vi "MeasureSinglePointAndStep.vi"(7 "SMU":T2, 8 "Error In":errorcluster, 9 "Source Value":dbl, 10 "Measure Function":T1, 11 "Keithley 2602 In":refnum<visa-resource-name>) -> (0 "Error Out":errorcluster, 2 "Reading":dbl, 3 "Keithley 2602 Out":refnum<visa-resource-name>)   [LabVIEW 2012, in "Keithley-2602.lvlib"]
uses:
  Keithley-2602.lvlib
  Controls/SMU.ctl
  Controls/MeasureFunction.ctl
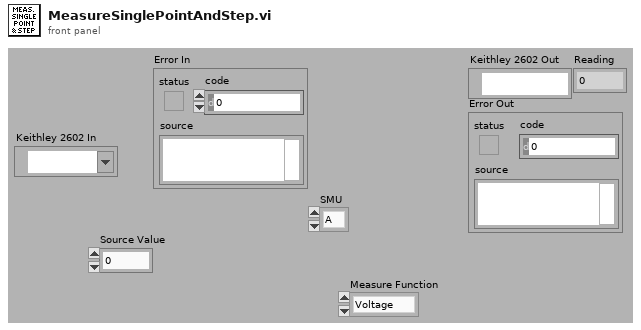
[diagram p1: front panel]
types:
  T1 = typedef "Keithley-2602.lvlib/MeasureFunction.ctl" = enum16{"Voltage", "Current", "Resistance", "Power"}
  T2 = typedef "Keithley-2602.lvlib/SMU.ctl" = enum16{"A", "B"}
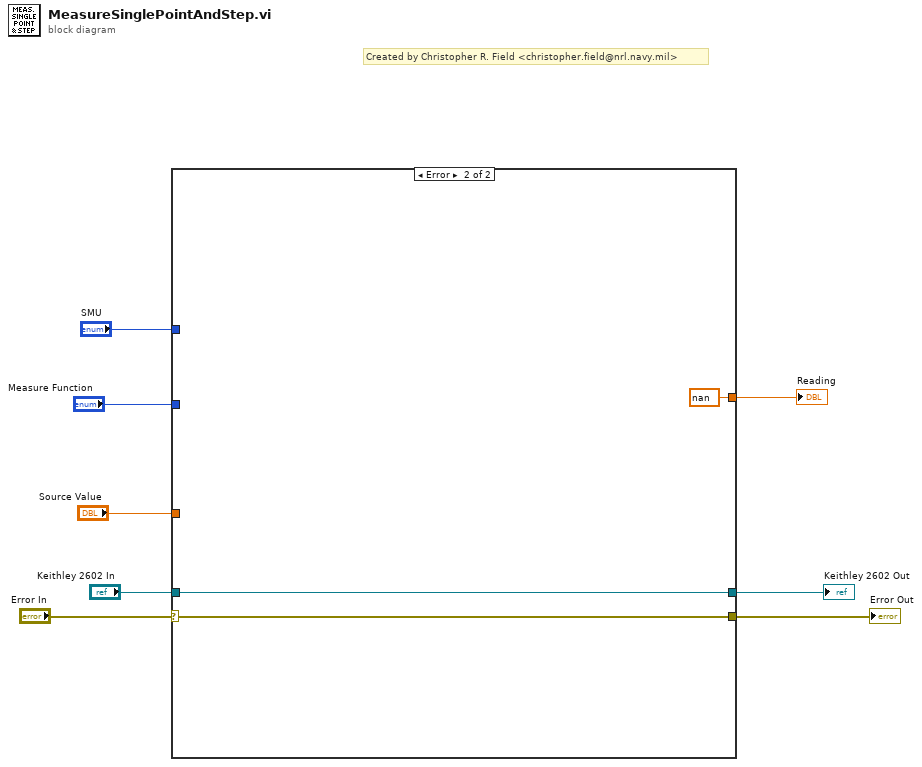
[diagram p0: block diagram]
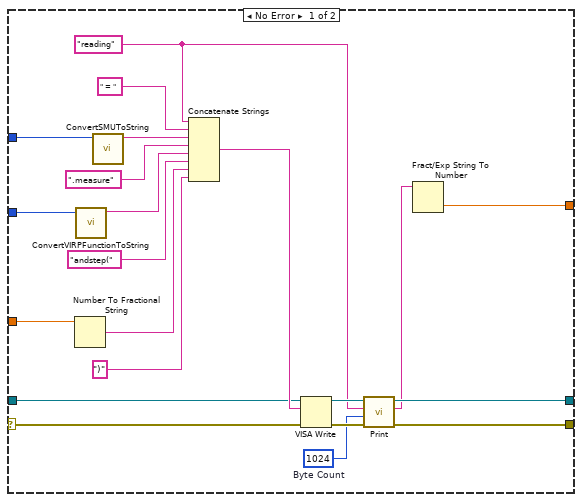
[diagram p2: hidden frame]
diagram:
  # "Created by Christopher R. Field <christopher.field@nrl.navy.mil>"
  n1 = case shown="Error" "Error In" {
    selector: "Error In" -> [w9 w31]
    tunnel: "Keithley 2602 In" -> [w23 w32]
    tunnel: [w18 w32] -> w7
    tunnel: [w17 w31] -> w6
    tunnel: [w15 nan] -> w5
    tunnel: "Source Value" -> [w14 _]
    tunnel: "SMU" -> [w11 _]
    tunnel: "Measure Function" -> [w10 _]
    frame No Error {
      w20 = u32 1024  # Byte Count
      w19 = "reading"
      n2 = Number To Fractional String(number=w14) -> (F-format string=w13:string)  [unwired: 3 in]
      n3 = call "ConvertVIRPFunctionToString.vi"("Function"=w10) -> ("Function"=w27:string)  [unwired: 10 in]
      n4 = call "ConvertSMUToString.vi"("SMU"=w11) -> ("Channel"=w29:string)  [unwired: 10 in]
      n5 = Concatenate Strings(w19, " = ", w29, ".measure", w27, "andstep(" ("string"), w13, ")" ("string")) -> (w24:string)
      n6 = VISA Write(VISA resource name=w23, write buffer=w24, error in (no error)=w9) -> (VISA resource name out=w22:refnum<visa-resource-name>, error out=w21:errorcluster)  [unwired: 1 out]
      n7 = call "Print.vi"("Error In"=w21, "Byte Count"=w20, "Attribute"=w19, "Kiethley 2602 In"=w22) -> ("Error Out"=w17:errorcluster, "Output"=w16:string, "Keithley 2602 Out"=w18:refnum<visa-resource-name>)  [unwired: 5 in]
      n8 = Fract/Exp String To Number(string=w16) -> (number=w15:dbl)  [unwired: 3 in, 1 out]
    }
    frame Error {
    }
  }
  "Keithley 2602 Out" <- w7
  "Error Out" <- w6
  "Reading" <- w5
